vi "example.vi"() -> ()   [LabVIEW 2018]
panel:
  in  "分頁":T1(tab)
  out "資料搜索結果":string[][](table)
  out "θX(左右) 2":cluster{timestamp[], dbl[]}(graph)
  out "θZ(前後) 2":cluster{timestamp[], dbl[]}(graph)
  out "θY(上下) 2":cluster{timestamp[], dbl[]}(graph)
  out "雨量 2":cluster{timestamp[], dbl[]}(graph)
  out "濕度 2":cluster{timestamp[], dbl[]}(graph)
  out "溫度 2":cluster{timestamp[], dbl[]}(graph)
  in  "最新資料查詢":bool
  out "最新資料查詢":string[][](table)
  out "時間":string
  out "時間":string
  out "時間":string
  out "時間":string
  out "θY(上下)":dbl
  out "θZ(前後)":dbl
  in  "stop":bool
  in  "結束時間":timestamp format="%<%Y%m%d >T"
  in  "開始時間":timestamp format="%<%Y%m%d >T"
  in  "進行查詢":bool
  in  "原始資料下載":bool
  out "日期":string
  out "日期":string
  out "?":string
  out "θX(左右)":dbl
  out "日期":string
  out "溫度":dbl
  out "日期":string
  out "濕度":dbl
  out "?":string
  out "?":string
  out "?":string
  out "雨量":dbl
  in  "Slide 4":dbl(slide) scale=0.0..10.0
  in  "Slide 4":dbl(slide) scale=0.0..10.0
  in  "Slide 4":dbl(slide) scale=0.0..10.0
  in  "Slide 4":dbl(slide) scale=0.0..10.0
  # "芳蘭社區"
  # "芳蘭社區"
  # "mm"
  # "RH"
  # "溼度"
  # "雨量"
  # "此處的資料會顯示您所選取的\"結束時間\"\n最後一筆資料的日期、時間、雨量、濕度、溫度與傾斜角"
  # "待觀察"
  # "待觀察"
  # "安全"
  # "需立即處理"
  # "安全"
  # "需立即處理"
  # "芳蘭社區"
  # "芳蘭社區"
  # "C"
  # "渡弊"
  # "溫度"
  # "待觀察"
  # "待觀察"
  # "安全"
  # "需立即處理"
  # "安全"
  # "需立即處理"
  # "分頁功能:\nMap:顯示芳蘭社區的Google地圖\n資料搜索結果:顯示從\"開始時間\"到\"結束時間\"範圍內所有的資料結果\nθX(左右):將\"資料搜索結果\"中θX的資料以圖形方式呈現\nθZ(前後):將\"資料搜索結果\"中θZ的資料以圖形方式呈現\nθY(上下):將\"資料搜索結果\"中θY的資料以圖形方式呈現\n雨量\"將\"資料搜索結果\"中雨量的資料以圖形方式呈現\n濕度\"將\"資料搜索結果\"中濕度的資料以圖形方式呈現\n溫度:將\"資料搜索結果\"中溫度的資料以圖形方式呈現\n最新資料查詢:按下\"最新資料查詢\"的綠色按鈕能夠顯示當前時間的最新一筆資料"
  # "按下\"原始資料下載\"，將\"資料搜索結果\"中的所有資料以excel方式儲存下來，\n路徑為builds > sheetAPI > My Application > CSV > CSV data"
  # "動態時間搜尋"
  # "開始時間"
  # "選取\"開始時間\"與\"結束時間\"的日期後，按下進行查詢，會將範圍內的資料顯示在\"資料搜索結果\"。\n開始時間的上限值為2023年5月9日下午 3:25，再往前的資料不會顯示出來。"
  # "結束時間"
  # "*註：若想搜尋任月份全部資料(如7月)，「開始時間」請輸入20180630，而「結束時間」請輸入20180801，也就是欲搜尋區段內再各加減一天，謝謝！"
  # "按下STOP按鈕\n停止執行程式"
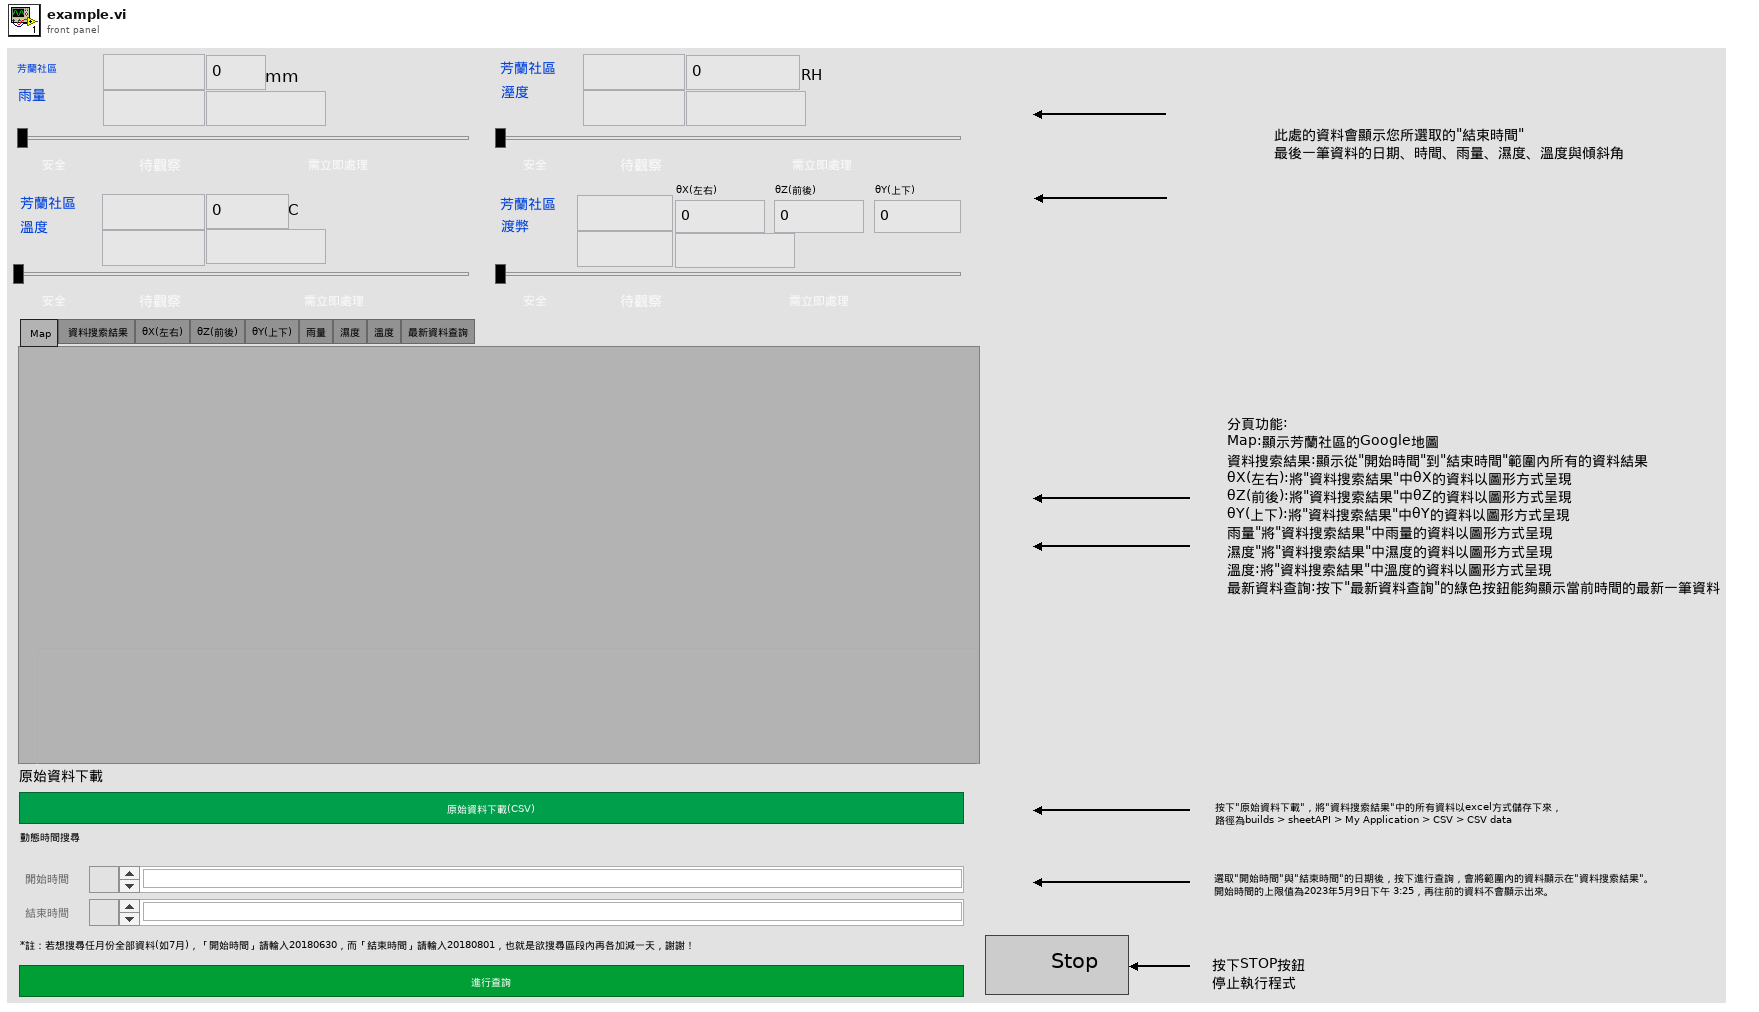
[diagram p1: front panel]
types:
  T1 = enum32{" Map", " 資料搜索結果", "θX(左右)", "θZ(前後)", "θY(上下)", "雨量", "濕度", "溫度", "最新資料查詢"}
  T2 = enum16{"open", "replace", "create", "open or create", "replace or create", "replace or create with confirmation"}
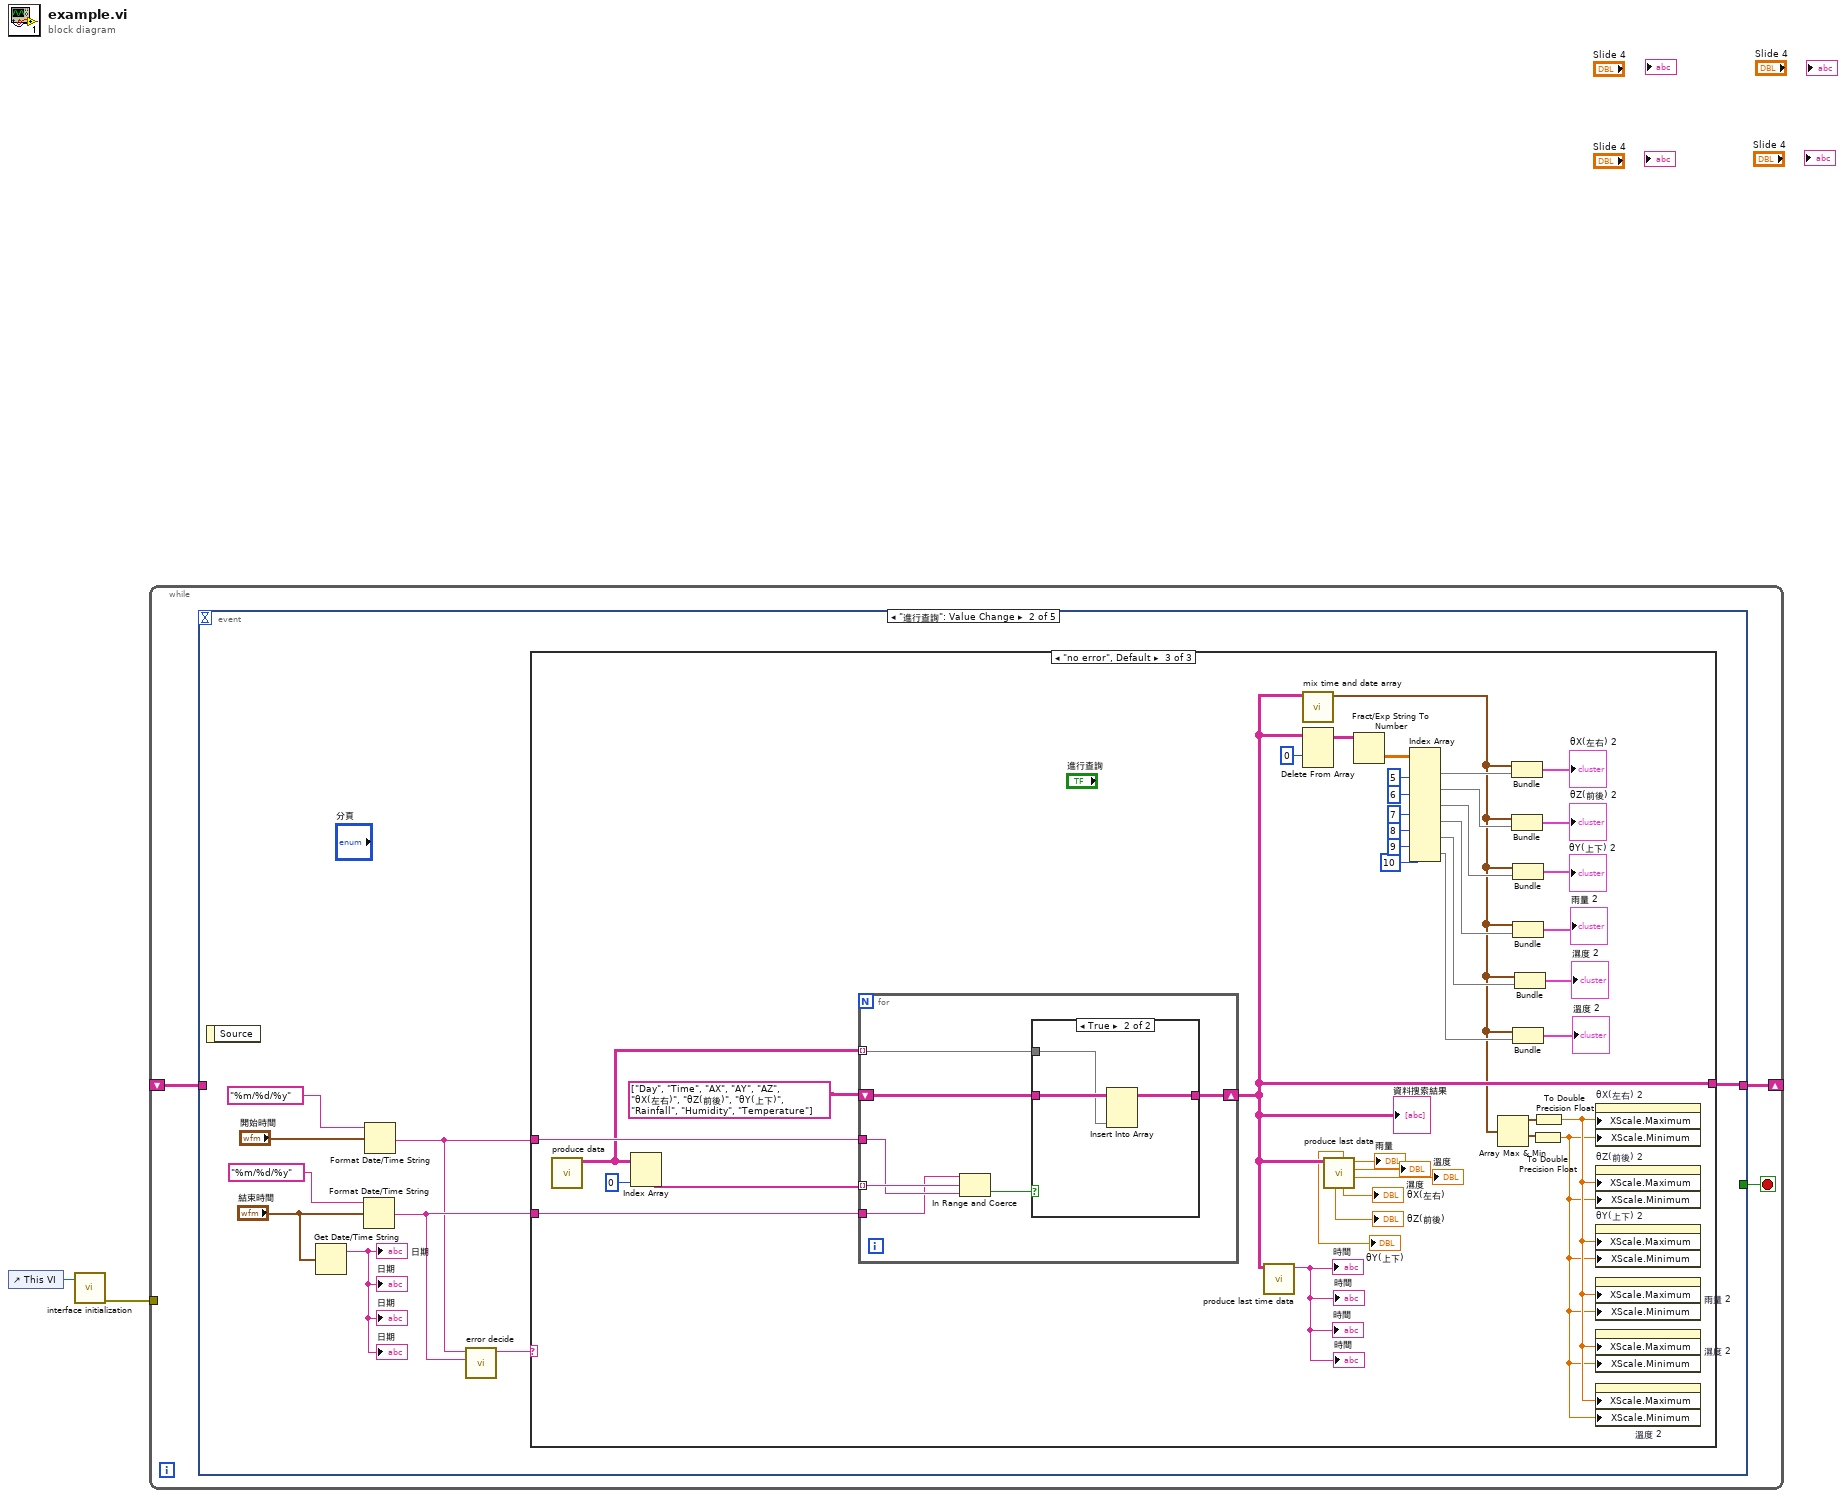
[diagram p0: block diagram]
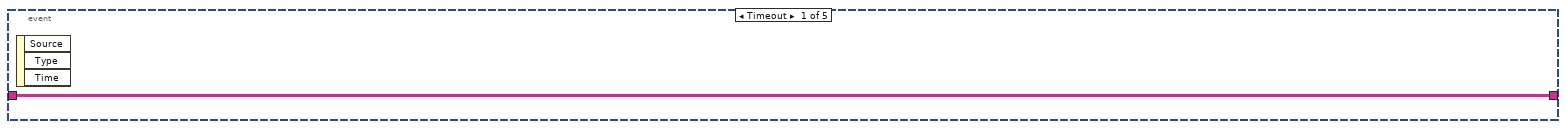
[diagram p2: hidden frame]
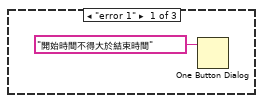
[diagram p3: hidden frame]
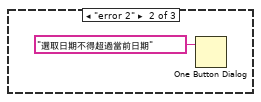
[diagram p4: hidden frame]
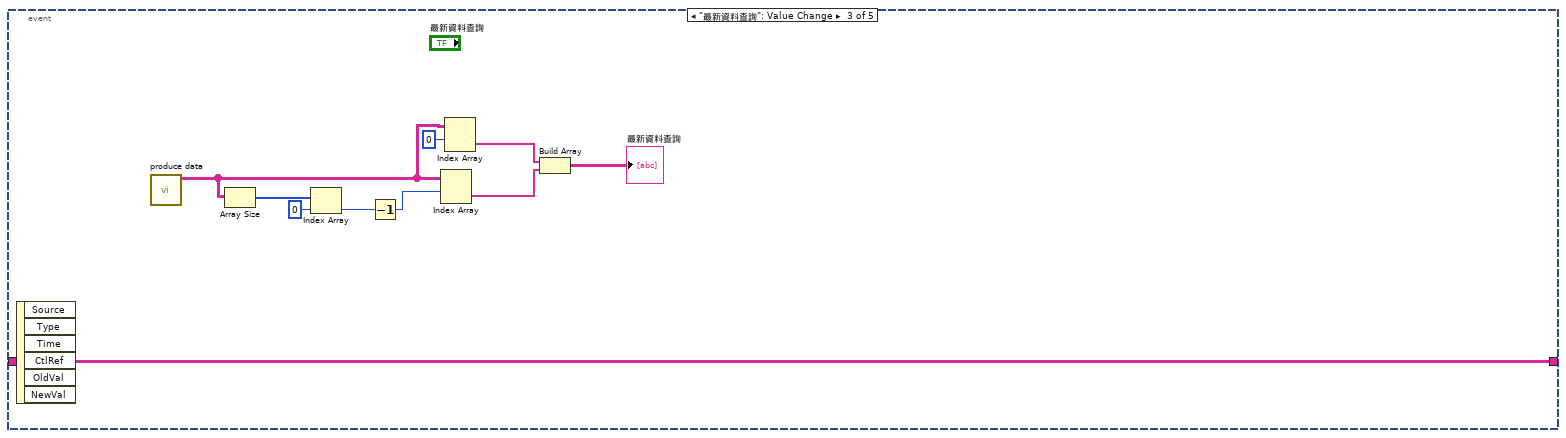
[diagram p6: hidden frame]
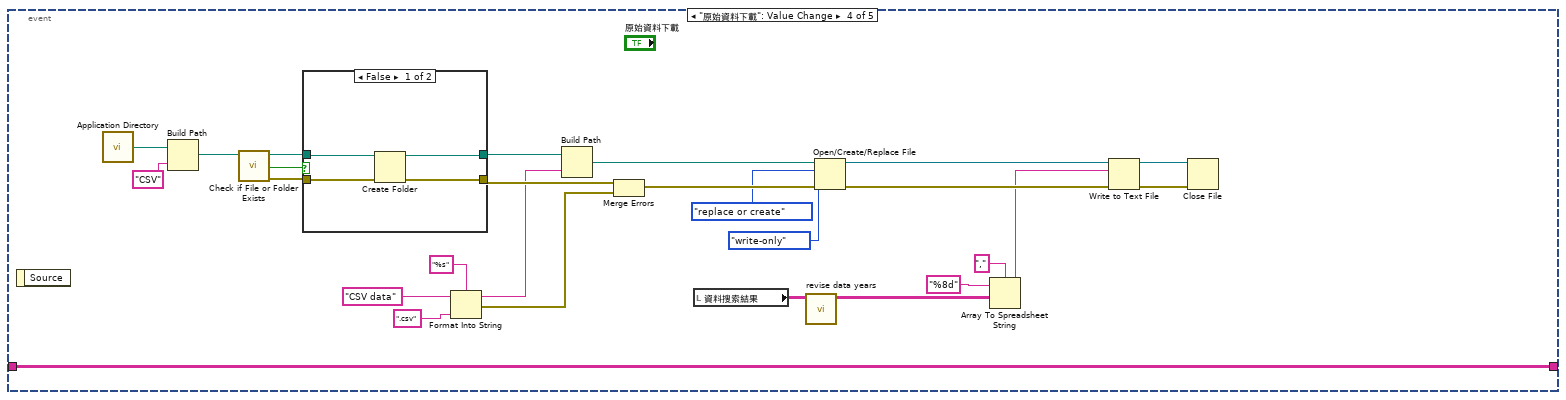
[diagram p7: hidden frame]
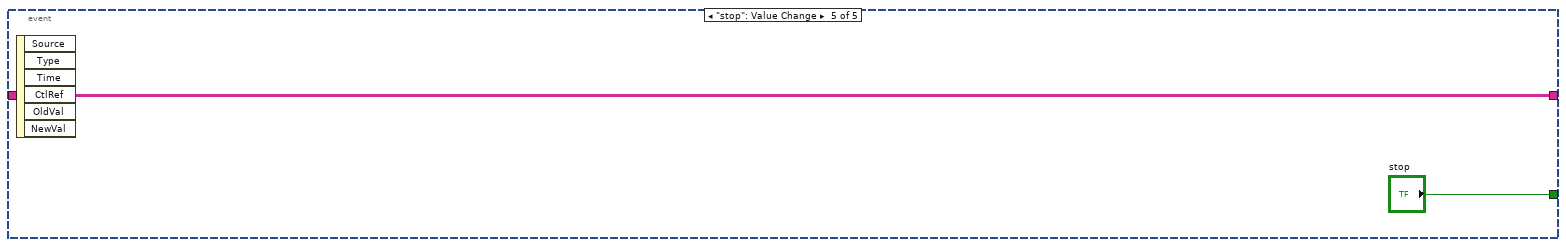
[diagram p9: hidden frame]
diagram:
  n1 = control-ref of="This VI"() -> (w2:refnum<vi>)
  n2 = call "interface initialization.vi"("VI in"=w2) -> ("error out"=w1:errorcluster)  [unwired: 10 in]
  n3 = while {
    shift-right: [w4] -> _
    shift-left: _ -> [w3]
    tunnel: w1 -> [_]
    stop <- w5 stop-if-true
    n4 = event shown="[1] \"進行查詢\": Value Change" {
      selector: _ -> [_ _ _ _ _]
      dyn-events: _ -> [_ _ _ _ _]
      timeout: _ -> [_ _ _ _ _]
      tunnel: [_ _ _ _ "stop"] -> w5
      tunnel: [w6 w9 w69 w79 w112] -> w4
      tunnel: w3 -> [w6 _ w69 w79 w112]
      event Timeout {
        n5 = event-data() -> ()  [unwired: 1 in, 3 out]
      }
      event "進行查詢": Value Change {
        n6 = event-data() -> ()  [unwired: 1 in, 1 out]
        n7 = Get Date/Time String(seconds (now)="結束時間") -> (date string=→"日期" →"日期" →"日期" →"日期":string)  [unwired: 2 in, 1 out]
        n8 = Format Date/Time String(time format string (%c)="%m/%d/%y", seconds (now)="結束時間") -> (date/time string=w8:string)  [unwired: 1 in]
        n9 = Format Date/Time String(time format string (%c)="%m/%d/%y", seconds (now)="開始時間") -> (date/time string=w7:string)  [unwired: 1 in]
        n10 = call "error decide.vi"("date/time string"=w8, "date/time string 2"=w7) -> ("String"=w12:string)  [unwired: 9 in]
        n11 = case shown="\"no error\", Default" w12 {
          tunnel: w7 -> [_ _ w52]
          tunnel: [_ _ w49] -> w9
          tunnel: w8 -> [_ _ w48]
          frame "error 1" {
            n12 = One Button Dialog(message="開始時間不得大於結束時間") -> ()  [unwired: 1 in, 1 out]
          }
          frame "error 2" {
            n13 = One Button Dialog(message="選取日期不得超過當前日期") -> ()  [unwired: 1 in, 1 out]
          }
          frame "no error", Default {
            n14 = call "produce data.vi"() -> ("res"=w51:string[][])  [unwired: 11 in]
            n15 = Index Array(array=w51, index (col)=0 ("disabled index (col)")) -> (element=w57:string[])  [unwired: 1 in]
            n16 = for {
              tunnel: w57 -> [w60] mode=indexing
              tunnel: w51 -> [w61] mode=indexing
              shift-right: [w62] -> w49
              shift-left: string[][] [["Day", "Time", "AX", "AY", "AZ", "θX(左右)", "θZ(前後)", "θY(上下)", "Rainfall", "Humidity", "Temperature"]] -> [w63]
              tunnel: w52 -> [w59]
              tunnel: w48 -> [w58]
              n17 = In Range and Coerce(upper limit=w58, x=w60, lower limit=w59) -> (In Range?=w64:bool)  [unwired: 1 out]
              n18 = case shown="True" w64 {
                tunnel: w63 -> [w65 w68]
                tunnel: [w65 w67] -> w62
                tunnel: w61 -> [_ w66]
                frame False {
                }
                frame True {
                  n19 = Insert Into Array(array=w68, new element=w66) -> (w67:string[][])  [unwired: 2 in]
                }
              }
            }
            "資料搜索結果" <- w49
            n20 = call "produce last time data.vi"("Array"=w49) -> ("String"=→"時間" →"時間" →"時間" →"時間":string)  [unwired: 10 in]
            n21 = call "mix time and date array.vi"("Array in"=w49) -> ("Array out"=w22:timestamp[])  [unwired: 10 in]
            n22 = Delete From Array(array=w49, index (row)=0) -> (array with subset deleted=w42:string[][])  [unwired: 2 in, 1 out]
            n23 = call "produce last data.vi"("Array"=w49) -> ("Numeric 4"=→"溫度":dbl, "Numeric 5"=→"濕度":dbl, "Numeric 6"=→"雨量":dbl, "Numeric 3"=→"θX(左右)":dbl, "Numeric"=→"θY(上下)":dbl, "Numeric 2"=→"θZ(前後)":dbl)  [unwired: 5 in]
            n24 = Fract/Exp String To Number(string=w42) -> (number=w41:dbl[][])  [unwired: 3 in, 1 out]
            n25 = Index Array(array=w41, index (col) #1=5 ("disabled index (col)"), index (col) #2=6 ("index (col)"), index (col) #3=7 ("index (col)"), index (col) #4=8 ("index (col)"), index (col) #5=9 ("index (col)"), index (col) #6=10 ("index (col)")) -> (element #1=w34:dbl[], element #2=w32:dbl[], element #3=w31:dbl[], element #4=w30:dbl[], element #5=w29:dbl[], element #6=w28:dbl[])  [unwired: 6 in]
            n26 = Array Max & Min(array=w22) -> (max value=w21:timestamp, min value=w20:timestamp)  [unwired: 2 out]
            n27 = Bundle("Array out"=w22, w34) -> (→"θX(左右) 2":cluster{"Array out":timestamp[], dbl[]})  [unwired: 1 in]
            n28 = Bundle("Array out"=w22, w32) -> (→"θZ(前後) 2":cluster{"Array out":timestamp[], dbl[]})  [unwired: 1 in]
            n29 = Bundle("Array out"=w22, w31) -> (→"θY(上下) 2":cluster{"Array out":timestamp[], dbl[]})  [unwired: 1 in]
            n30 = Bundle("Array out"=w22, w30) -> (→"雨量 2":cluster{"Array out":timestamp[], dbl[]})  [unwired: 1 in]
            n31 = Bundle("Array out"=w22, w28) -> (→"溫度 2":cluster{"Array out":timestamp[], dbl[]})  [unwired: 1 in]
            n32 = Bundle("Array out"=w22, w29) -> (→"濕度 2":cluster{"Array out":timestamp[], dbl[]})  [unwired: 1 in]
            n33 = To Double Precision Float(number=w20) -> (double precision float=w18:dbl)
            n34 = To Double Precision Float(number=w21) -> (double precision float=w19:dbl)
            n35 = property on="θX(左右) 2" class="XYGraph (strict)"("XScale.Maximum"=w19, "XScale.Minimum"=w18) -> ()  [unwired: 2 in, 2 out]
            n36 = property on="θZ(前後) 2" class="XYGraph (strict)"("XScale.Maximum"=w19, "XScale.Minimum"=w18) -> ()  [unwired: 2 in, 2 out]
            n37 = property on="θY(上下) 2" class="XYGraph (strict)"("XScale.Maximum"=w19, "XScale.Minimum"=w18) -> ()  [unwired: 2 in, 2 out]
            n38 = property on="雨量 2" class="XYGraph (strict)"("XScale.Maximum"=w19, "XScale.Minimum"=w18) -> ()  [unwired: 2 in, 2 out]
            n39 = property on="濕度 2" class="XYGraph (strict)"("XScale.Maximum"=w19, "XScale.Minimum"=w18) -> ()  [unwired: 2 in, 2 out]
            n40 = property on="溫度 2" class="XYGraph (strict)"("XScale.Maximum"=w19, "XScale.Minimum"=w18) -> ()  [unwired: 2 in, 2 out]
          }
        }
      }
      event "最新資料查詢": Value Change {
        n41 = event-data() -> ()  [unwired: 1 in, 6 out]
        n42 = call "produce data.vi"() -> ("res"=w70:string[][])  [unwired: 11 in]
        n43 = Array Size(array=w70) -> (size(s)=w75:i32[])
        n44 = Index Array(array=w75, index=0) -> (element=w74:i32)
        n45 = Decrement(x=w74) -> (x-1=w77:i32)
        n46 = Index Array(array=w70, index (row)=w77) -> (element=w72:string[])  [unwired: 1 in]
        n47 = Index Array(array=w70, index (row)=0) -> (element=w73:string[])  [unwired: 1 in]
        n48 = Build Array(w73, w72) -> (→"最新資料查詢":string[][])
      }
      event "原始資料下載": Value Change {
        n49 = event-data() -> ()  [unwired: 1 in, 1 out]
        n50 = call <vilib>:"Application Directory.vi"() -> ("Application Directory"=w105:path)
        n51 = Build Path(base path=w105, name or relative path="CSV") -> (appended path=w103:path)
        n52 = call <vilib>:"Check if File or Folder Exists.vi"("path"=w103) -> ("error out"=w100:errorcluster, "file or folder exists?"=w102:bool, "dup path"=w101:path)  [unwired: 8 in]
        n53 = case shown="False" w102 {
          tunnel: w101 -> [w109 w111]
          tunnel: w100 -> [w108 w110]
          tunnel: [w107 w111] -> w99
          tunnel: [w106 w110] -> w86
          frame False {
            n54 = Create Folder(path (use dialog)=w109, error in=w108) -> (created path=w107:path, error out=w106:errorcluster)  [unwired: 1 in, 1 out]
          }
          frame True {
          }
        }
        n55 = Format Into String(format string="%s", initial string="CSV data", ".csv" ("input 1")) -> (resulting string=w84:string, error out=w85:errorcluster)  [unwired: 1 in]
        n56 = Build Path(base path=w99, name or relative path=w84) -> (appended path=w98:path)
        n57 = Merge Errors(w86, w85) -> (w87:errorcluster)
        n58 = local read "資料搜索結果"() -> (w80:string[][])
        n59 = call "revise data years.vi"("Array in"=w80) -> ("Array out"=w81:string[][])  [unwired: 10 in]
        n60 = Open/Create/Replace File(file path (use dialog)=w98, error in=w87, operation (0:open)=T2."replace or create", access (0:read/write)=enum16{"read/write", "read-only", "write-only"}."write-only") -> (refnum out=w92:refnum<file>, error out=w89:errorcluster)  [unwired: 2 in, 1 out]
        n61 = Array To Spreadsheet String(delimiter (Tab)=",", array=w81, 3:"%8d" ("format string")) -> (spreadsheet string=w88:string)
        n62 = Write to Text File(file (use dialog)=w92, text=w88, error in=w89) -> (refnum out=w91:refnum<file>, error out=w90:errorcluster)  [unwired: 1 in, 1 out]
        n63 = Close File(refnum=w91, error in=w90) -> ()  [unwired: 2 out]
      }
      event "stop": Value Change {
        n64 = event-data() -> ()  [unwired: 1 in, 6 out]
      }
    }
  }
